vi "Read exeRef.vi"(8 "error in (no error)":errorcluster, 11 "LT_UpgradeFlash in":refnum<class "LT_UpgradeFlash.lvclass">) -> (0 "error out":errorcluster, 2 "exeRef":refnum<k24>, 3 "LT_UpgradeFlash out":refnum<class "LT_UpgradeFlash.lvclass">)   [LabVIEW 2017, in "LT_UpgradeFlash.lvclass"]
uses:
  LT_UpgradeFlash.lvclass
  D:/Project/Tymphany/LT_UpgradeFlash/LT_UpgradeFlash_dll/LT_UpgradeFlash_dll/bin/Debug/LT_UpgradeFlash_dll.dll
  LT_UpgradeFlash_dll/LT_UpgradeFlash_dll/bin/Debug/LT_UpgradeFlash_dll.dll
  LT_UpgradeFlash.lvclass/LT_UpgradeFlash.ctl
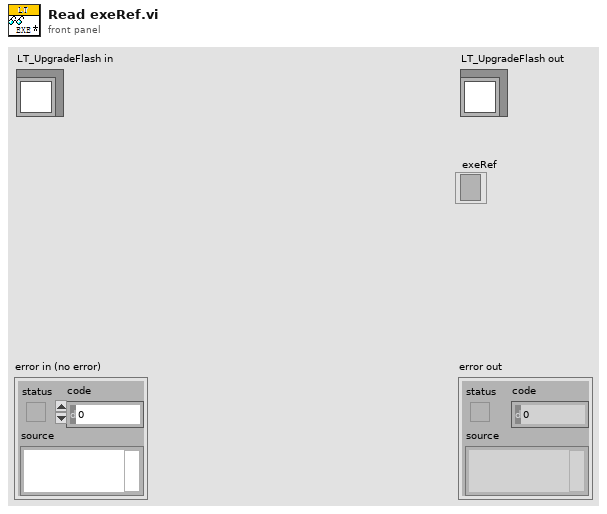
[diagram p1: front panel]
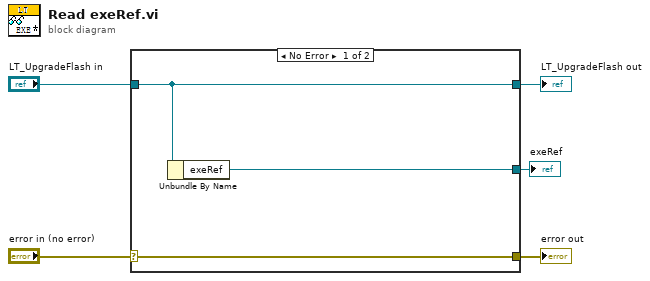
[diagram p0: block diagram]
diagram:
  n1 = case shown="No Error" "error in (no error)" {
    selector: "error in (no error)" -> [w8 w9]
    tunnel: [w8 w9] -> w4
    tunnel: [w7 w10] -> w2
    tunnel: "LT_UpgradeFlash in" -> [w7 w10]
    tunnel: [w6 _] -> w1
    frame No Error {
      n2 = Unbundle By Name(w7) -> ("exeRef"=w6:refnum<k24>)
    }
    frame Error {
    }
  }
  "error out" <- w4
  "LT_UpgradeFlash out" <- w2
  "exeRef" <- w1
